vi "midterm.vi"() -> ()   [LabVIEW 2009]
panel:
  in  "Stop Pressed":bool
  in  "Enter Password":string
  out "Arm Countdown":i32
  out "Front door indicator":bool[](array[boolean])
  out "Alarm Countdown":i32
  out "Alarm":bool
  out "On indicates open":bool[](array[boolean])
  in  "Disarm":bool
  out "Armed":bool
  in  "?":bool
  # "Burglar Alarm System"
  # "Window 1"
  # "Window 2"
  # "Back door"
  # "Front door"
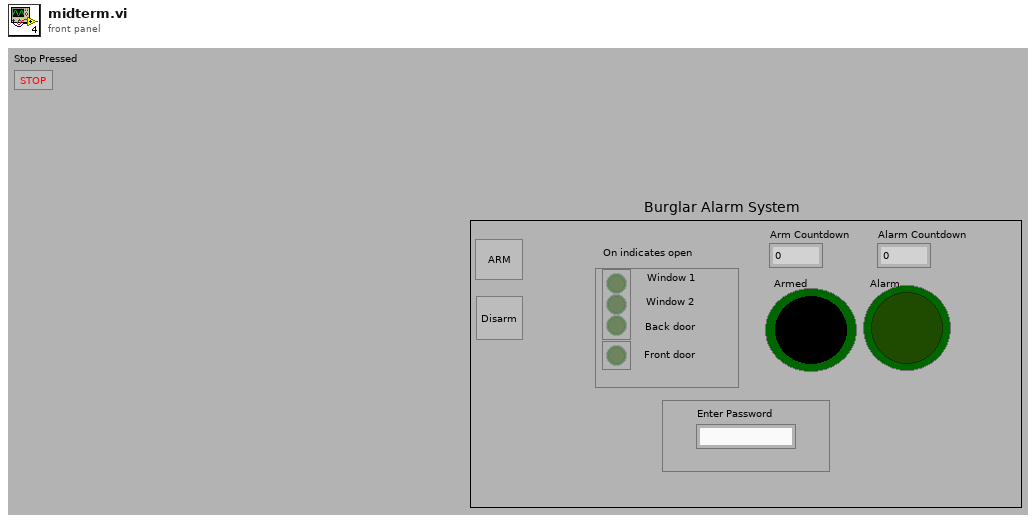
[diagram p1: front panel]
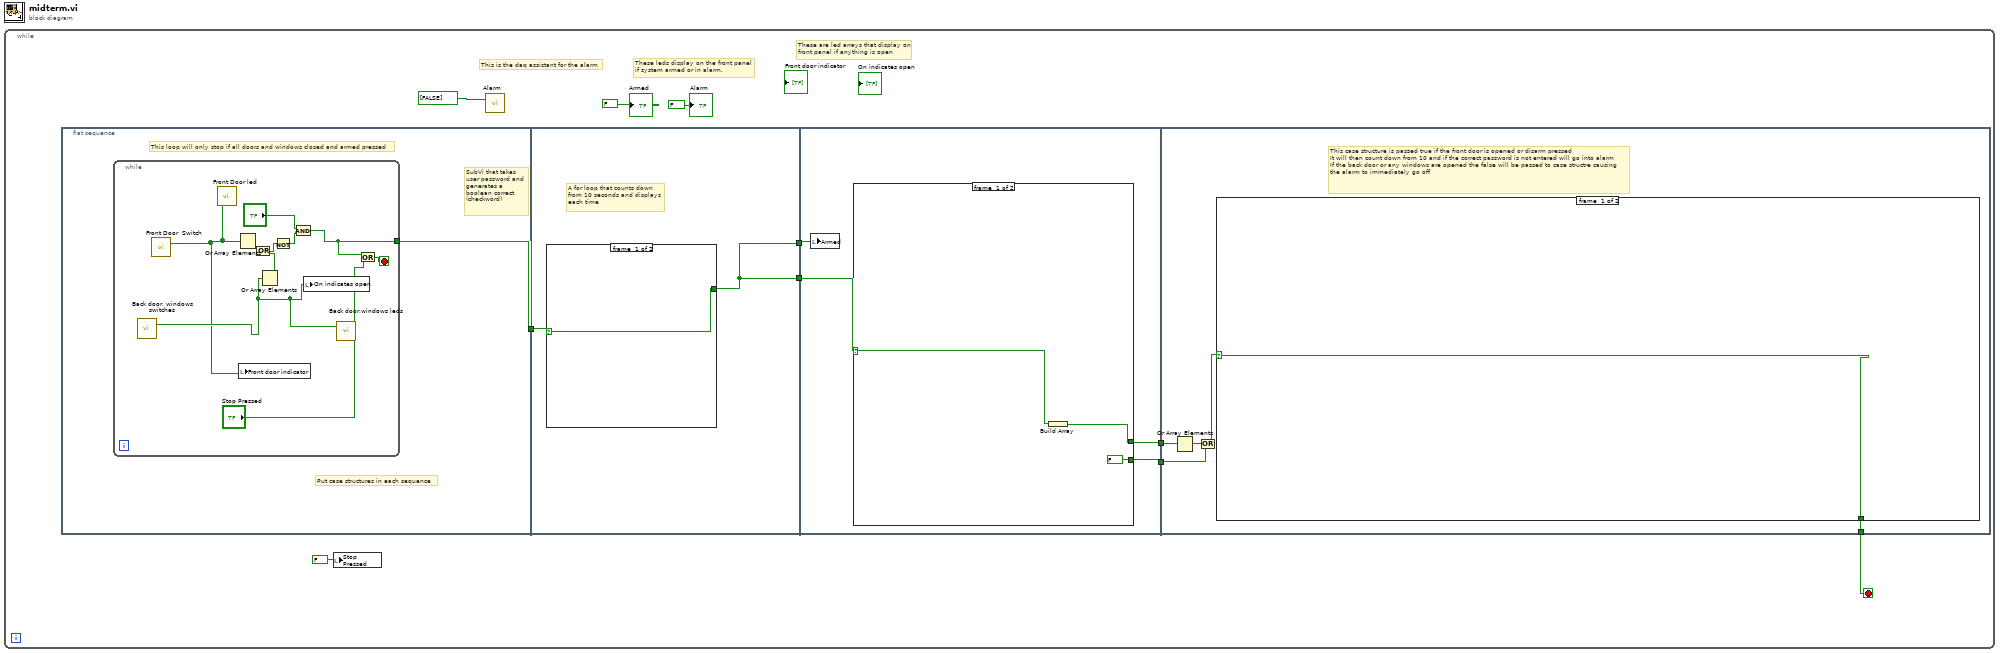
[diagram p0: block diagram]
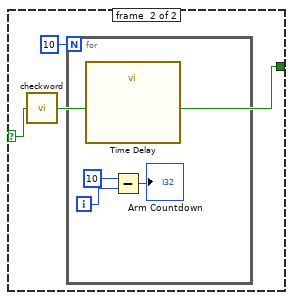
[diagram p2: hidden frame]
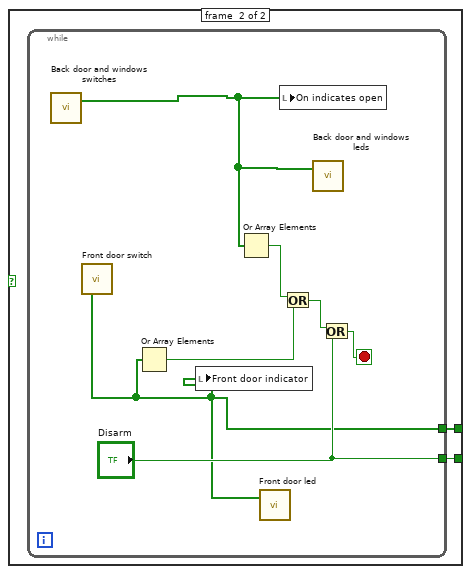
[diagram p3: hidden frame]
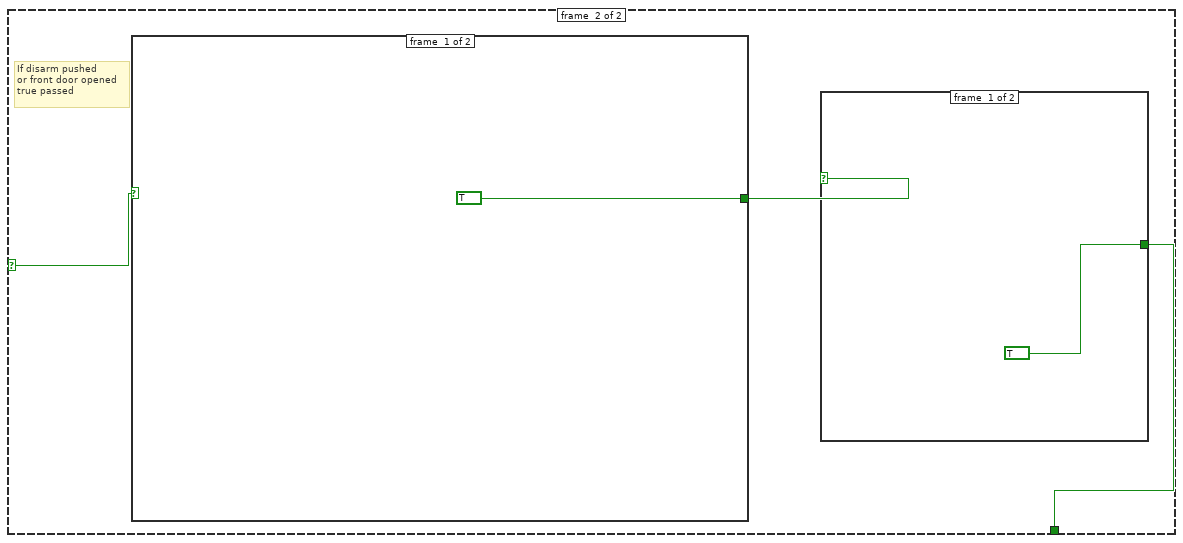
[diagram p4: hidden frame]
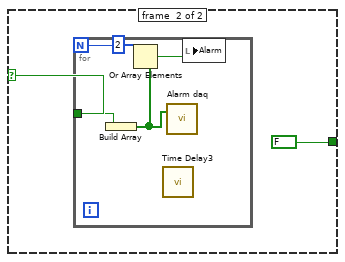
[diagram p5: hidden frame]
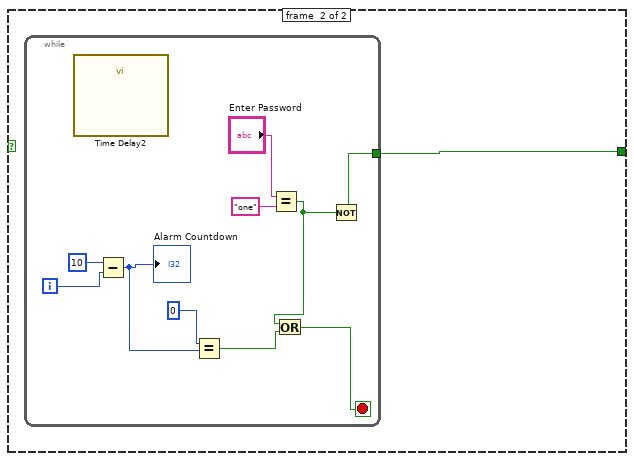
[diagram p6: hidden frame]
diagram:
  n1 = while {
    stop <- w1 stop-if-true
    # "This is the daq assistant for the alarm"
    # "These are led arrays that display on\nfront panel if anything is open"
    # "These leds display on the front panel\nif system armed or in alarm."
    n2 = flat-sequence {
      tunnel: [w11] -> w4
      tunnel: [w22] -> w5
      tunnel: w4 -> [w23]
      tunnel: [w22] -> w3
      tunnel: [w34] -> w10
      tunnel: [w33] -> w9
      tunnel: w5 -> [w32]
      tunnel: w3 -> [w31]
      tunnel: w10 -> [w51]
      tunnel: w9 -> [w49]
      tunnel: [w47] -> w1
      frame #0 {
        # "Put case structures in each sequence"
        # "SubVi that takes user password and \ngenerates a boolean correct\n(checkword)"
        # "This loop will only stop if all doors and windows closed and armed pressed"
        n3 = while {
          tunnel: [w13] -> w11
          stop <- w12 stop-if-true
          n4 = call "Back door, windows switches"() -> ("data"=w16:bool[])  [unwired: 17 in, 2 out]
          n5 = call "Front Door  Switch"() -> ("data"=w15:bool[])  [unwired: 17 in, 2 out]
          n6 = call "Front Door led"("data"=w15) -> ()  [unwired: 17 in, 2 out]
          n7 = Or Array Elements(Boolean array=w15) -> (logical OR=w19:bool)
          n8 = local write "Front door indicator"(w15) -> ()
          n9 = Or Array Elements(Boolean array=w16) -> (logical OR=w18:bool)
          n10 = Or(x=w19, y=w18) -> (x .or. y?=w17:bool)
          n11 = Not(x=w17) -> (.not. x?=w20:bool)
          n12 = And(x="?", y=w20) -> (x .and. y?=w13:bool)
          n13 = local write "On indicates open"(w16) -> ()
          n14 = call "Back door,windows leds"("data"=w16) -> ()  [unwired: 17 in, 2 out]
          n15 = Or(x=w13, y="Stop Pressed") -> (x .or. y?=w12:bool)
        }
      }
      frame #1 {
        # "A for loop that counts down\nfrom 10 seconds and displays\neach time"
        n16 = case shown="True" w23 {
          selector: w23 -> [w24 w26]
          tunnel: [w24 w25] -> w22
          frame #0 {
          }
          frame #1 {
            n17 = call "checkword.vi"("Enable"=w26) -> ("Boolean"=w25:bool)
            n18 = for {
              N: 10 -> [_]
              i -> [w30]
              n19 = call "Time Delay"() -> ()  [unwired: 11 in, 1 out]
              n20 = Subtract(x=10, y=w30) -> (x-y=→"Arm Countdown":i32)
            }
          }
        }
      }
      frame #2 {
        n21 = local write "Armed"(w32) -> ()
        n22 = case shown="True" w31 {
          selector: w31 -> [w37 _]
          tunnel: [w36 w39] -> w34
          tunnel: [FALSE ("Disarm") w38] -> w33
          frame #0 {
            n23 = Build Array(w37) -> (w36:bool[])
          }
          frame #1 {
            n24 = while {
              tunnel: [w40] -> w39
              tunnel: ["Disarm"] -> w38
              stop <- w43 stop-if-true
              n25 = call "Back door and windows switches"() -> ("data"=w41:bool[])  [unwired: 17 in, 2 out]
              n26 = call "Front door switch"() -> ("data"=w40:bool[])  [unwired: 17 in, 2 out]
              n27 = Or Array Elements(Boolean array=w40) -> (logical OR=w45:bool)
              n28 = local write "Front door indicator"(w40) -> ()
              n29 = Or Array Elements(Boolean array=w41) -> (logical OR=w46:bool)
              n30 = call "Front door led"("data"=w40) -> ()  [unwired: 17 in, 2 out]
              n31 = local write "On indicates open"(w41) -> ()
              n32 = Or(x=w46, y=w45) -> (x .or. y?=w44:bool)
              n33 = call "Back door and windows leds"("data"=w41) -> ()  [unwired: 17 in, 2 out]
              n34 = Or(x=w44, y="Disarm") -> (x .or. y?=w43:bool)
            }
          }
        }
      }
      frame #3 {
        # "This case structure is passed true if the front door is opened or disarm pressed\nIt will then count down from 10 and if the correct password is not entered will go into alarm\nIf the back door or any windows are opened the false will be passed to case structre causing \nthe alarm to immediately go off"
        n35 = Or Array Elements(Boolean array=w51) -> (logical OR=w50:bool)
        n36 = Or(x=w49, y=w50) -> (x .or. y?=w48:bool)
        n37 = case shown="True" w48 {
          selector: w48 -> [w52 w54]
          tunnel: [w52 w53] -> w47
          frame #0 {
          }
          frame #1 {
            # "If disarm pushed\nor front door opened\ntrue passed"
            n38 = case shown="True" w54 {
              tunnel: [TRUE ("Alarm") w64] -> w55
              frame #0 {
              }
              frame #1 {
                n39 = while {
                  tunnel: [w65] -> w64
                  i -> [w74]
                  stop <- w67 stop-if-true
                  n40 = call "Time Delay2"() -> ()  [unwired: 11 in, 1 out]
                  n41 = Subtract(x=10, y=w74) -> (x-y=w72:i32)
                  "Alarm Countdown" <- w72
                  n42 = Equal?(x=0, y=w72) -> (x = y?=w68:bool)
                  n43 = Equal?(x="Enter Password", y="one") -> (x = y?=w66:bool)
                  n44 = Or(x=w66, y=w68) -> (x .or. y?=w67:bool)
                  n45 = Not(x=w66) -> (.not. x?=w65:bool)
                }
              }
            }
            n46 = case shown="True" w55 {
              selector: w55 -> [_ w58]
              tunnel: [TRUE ("Stop Program") FALSE ("Stop Program")] -> w53
              frame #0 {
              }
              frame #1 {
                n47 = for {
                  N: 2 -> [_]
                  tunnel: w58 -> [w61]
                  n48 = Build Array(w61) -> (w60:bool[])
                  n49 = Or Array Elements(Boolean array=w60) -> (logical OR=w62:bool)
                  n50 = call "Time Delay3"() -> ()  [unwired: 11 in, 1 out]
                  n51 = call "Alarm daq"("data"=w60) -> ()  [unwired: 17 in, 2 out]
                  n52 = local write "Alarm"(w62) -> ()
                }
              }
            }
          }
        }
      }
    }
    n53 = local write "Stop Pressed"(FALSE ("Stop Pressed")) -> ()
    n54 = call "Alarm"("data"=bool[] [FALSE]) -> ()  [unwired: 17 in, 2 out]
    "Armed" <- FALSE ("Armed")
    "Alarm" <- FALSE ("Alarm")
  }
